vi "WAIT.vi"(10 "argv":string[](array[string]), 11 "args":u8) -> ()   [LabVIEW 2015]
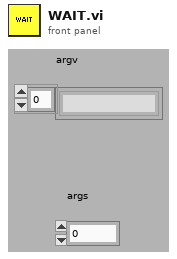
[diagram p1: front panel]
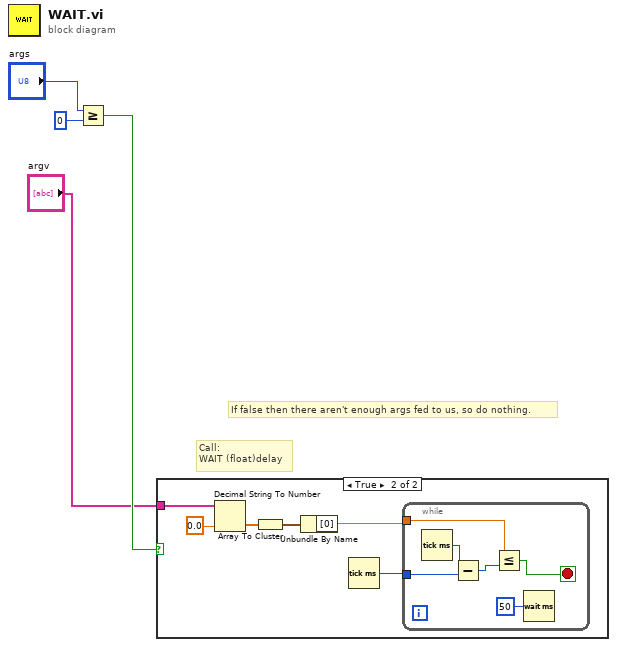
[diagram p0: block diagram]
diagram:
  # "If false then there aren't enough args fed to us, so do nothing."
  # "Call:\nWAIT (float)delay"
  n1 = Greater Or Equal?(x="args", y=u8 0) -> (x >= y?=w4:bool)
  n2 = case shown="True" w4 {
    tunnel: "argv" -> [_ w7]
    frame False {
    }
    frame True {
      n3 = Decimal String To Number(string=w7, default (0L)=0.0 ("default (0 I32)")) -> (number=w9:dbl[])  [unwired: 2 out]
      n4 = Array To Cluster(array=w9) -> (cluster=w8:cluster{"[0]":dbl, "[1]":dbl})
      n5 = Unbundle By Name(w8) -> ("[0]"=w6:dbl)
      n6 = Tick Count (ms)() -> (millisecond timer value=w5:u32)
      n7 = while {
        tunnel: w6 -> [w12]
        tunnel: w5 -> [w14]
        stop <- w11 stop-if-true
        n8 = Tick Count (ms)() -> (millisecond timer value=w15:u32)
        n9 = Subtract(x=w15, y=w14) -> (x-y=w13:u32)
        n10 = Less Or Equal?(x=w12, y=w13) -> (x <= y?=w11:bool)
        n11 = Wait (ms)(milliseconds to wait=u32 50) -> ()  [unwired: 1 out]
      }
    }
  }
